vi "POSTImgData.vi"(7 "base path":path, 8 "URL":string, 9 "name or relative path":string, 10 "image data":T1, 11 "unique experiment identifier":string) -> (0 "error out":errorcluster)   [LabVIEW 2016]
uses:
  <vilib>/picture/picture.llb/imagedata.ctl
  <vilib>/httpClient/MultipartData.ctl
  <vilib>/httpClient/LabVIEWHTTPClient.lvlib
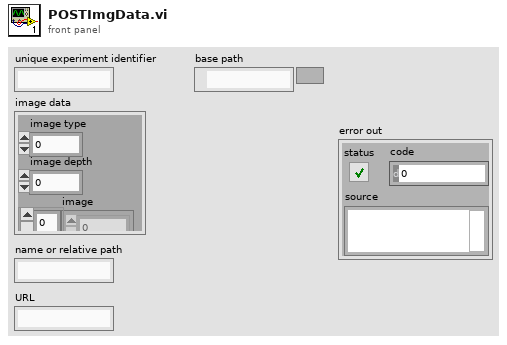
[diagram p1: front panel]
types:
  T1 = typedef "imagedata.ctl" = cluster{"image type":i32, "image depth":i32, "image":u8[], "mask":u8[], "colors":u32[], "Rectangle":cluster{"left":i16, "top":i16, "right":i16, "bottom":i16}}
  T2 = typedef "LabVIEWHTTPClient.lvlib/MultipartData.ctl" = cluster{"Name":string, "Value":string, "File":path, "Filename":string, "MIME type":string}
  T3 = typedef "LabVIEWHTTPClient.lvlib/ClientHandle.ctl" = refnum<k1>
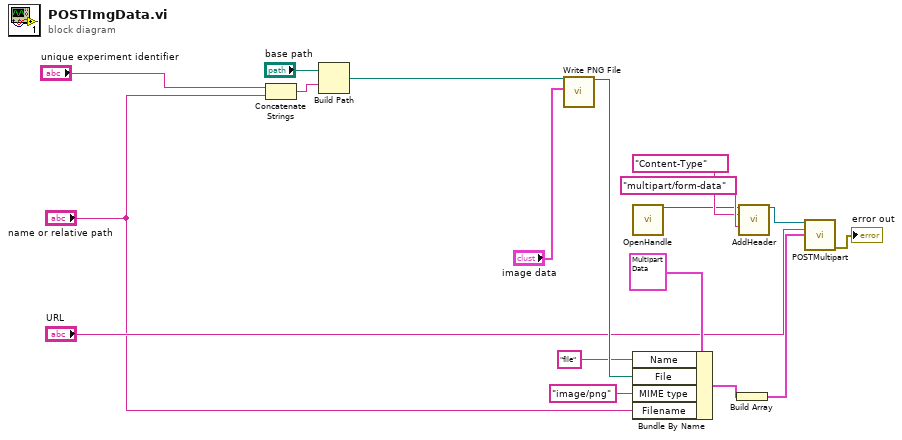
[diagram p0: block diagram]
diagram:
  n1 = Concatenate Strings("unique experiment identifier", "name or relative path") -> (w5:string)
  n2 = Build Path(base path="base path", name or relative path=w5) -> (appended path=w4:path)
  n3 = call <vilib>:"Write PNG File.vi"("image data"="image data", "path to PNG file"=w4) -> ("path"=w17:path)  [unwired: 8 in, 1 out]
  n4 = call <vilib>:"OpenHandle.vi"() -> ("client handle out"=w9:T3)  [unwired: 14 in, 1 out]
  n5 = Bundle By Name(cluster=T2 {"Name"="", "Value"="", "File"=path "", "Filename"="", "MIME type"="application/octet-stream"} ("Element"), "Name"="file", "File"=w17, "MIME type"="image/png", "Filename"="name or relative path") -> (w16:T2)
  n6 = Build Array(w16) -> (w18:T2[])
  n7 = call <vilib>:"AddHeader.vi"("client handle"=w9, "header"="Content-Type", "value"="multipart/form-data") -> ("client handle out"=w8:T3)  [unwired: 11 in, 1 out]
  n8 = call <vilib>:"POSTMultipart.vi"("client handle"=w8, "url"="URL", "data"=w18) -> ("error out"=→"error out":errorcluster)  [unwired: 9 in, 3 out]
